vi "Read Voltage Limits.vi"   [LabVIEW 2023, in "Voltage Limits.lvclass"]
uses:
  Voltage Limits.lvclass
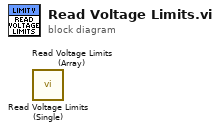
[diagram p0: block diagram]
diagram:
  n1 = call "Read Voltage Limits (Single).vi"() -> ()  [unwired: 7 in, 5 out]
  n2 = call "Read Voltage Limits (Array).vi"() -> ()  [unwired: 7 in, 5 out]
